vi "TEST Monitor Polling.vi"() -> ()   [LabVIEW 2013, in "C37118-DLL.lvlib"]
uses:
  C37118-DLL.lvlib
panel:
  out "Data?":bool
  in  "Poll Timeout":i32
  out "Delay":u32(graph)
  in  "milliseconds to wait":u32
  in  "stop":bool
  # "Test the data polling function"
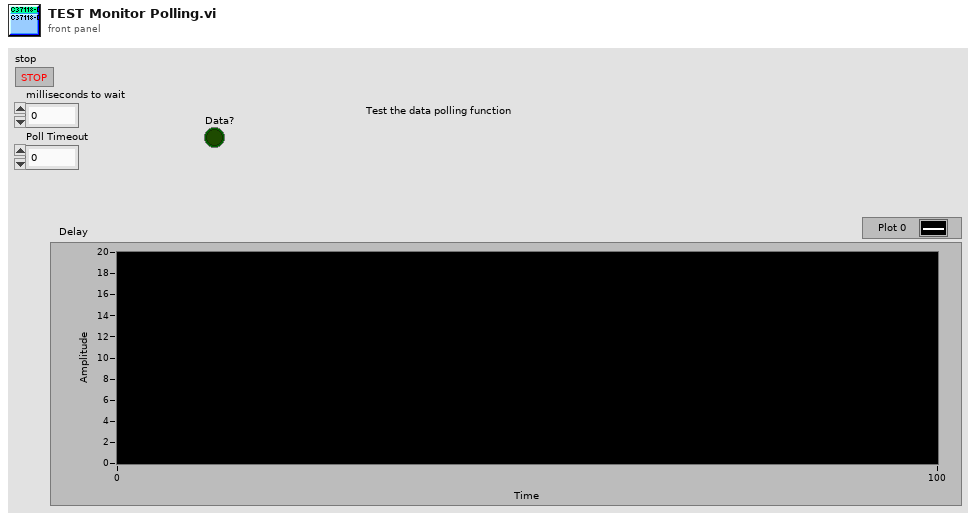
[diagram p1: front panel]
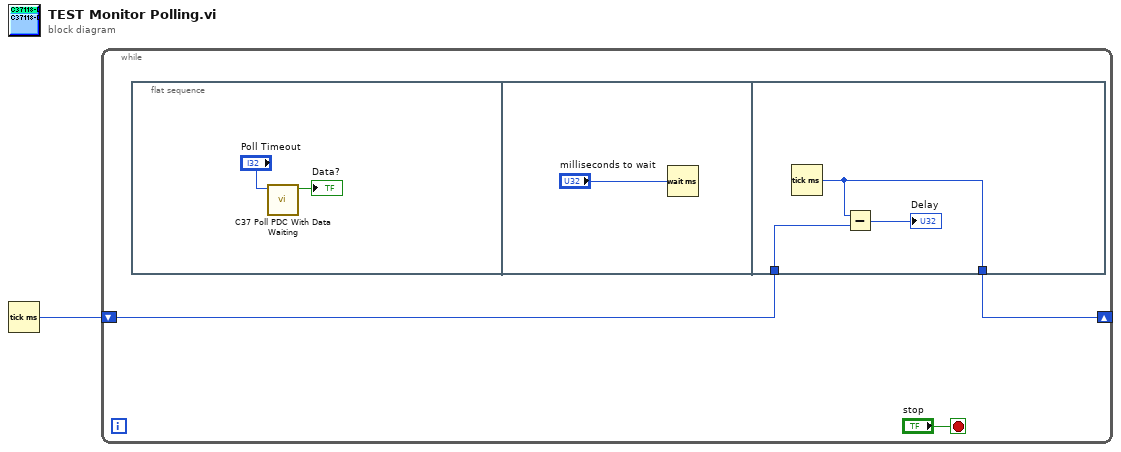
[diagram p0: block diagram]
diagram:
  n1 = Tick Count (ms)() -> (millisecond timer value=w1:u32)
  n2 = while {
    shift-right: [w2] -> _
    shift-left: w1 -> [w3]
    stop <- "stop" stop-if-true
    n3 = flat-sequence {
      tunnel: w3 -> [w9]
      tunnel: [w10] -> w2
      frame #0 {
        n4 = call "C37 Poll PDC With Data Waiting.vi"("Pseudo PDC ID"="Poll Timeout") -> ("Data?"=→"Data?":bool)  [unwired: 9 in, 1 out]
      }
      frame #1 {
        n5 = Wait (ms)(milliseconds to wait="milliseconds to wait") -> ()  [unwired: 1 out]
      }
      frame #2 {
        n6 = Tick Count (ms)() -> (millisecond timer value=w10:u32)
        n7 = Subtract(x=w10, y=w9) -> (x-y=→"Delay":u32)
      }
    }
  }
